vi "read_attributes.vi"(8 "error in (no error)":errorcluster, 11 "SVC in":refnum<class "SVC.lvclass">) -> (0 "error out":errorcluster, 2 "attributes":T1, 3 "SVC out":refnum<class "SVC.lvclass">)   [LabVIEW 2020, in "SVC.lvclass"]
uses:
  SVC.lvclass
  Controls/svc_attributes.ctl
  SVC.lvclass/SVC.ctl
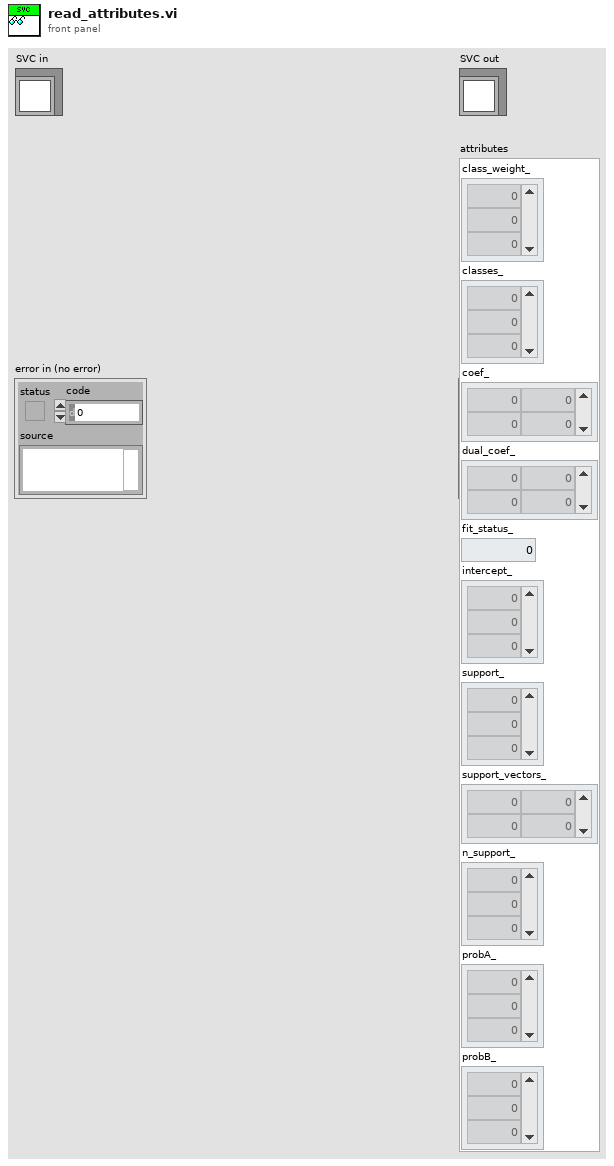
[diagram p1: front panel]
types:
  T1 = typedef "svc_attributes.ctl" = cluster{"class_weight_":dbl[], "classes_":dbl[], "coef_":dbl[][], "dual_coef_":dbl[][], "fit_status_":dbl, "intercept_":dbl[], "support_":dbl[], "support_vectors_":dbl[][], "n_support_":dbl[], "probA_":dbl[], "probB_":dbl[]}
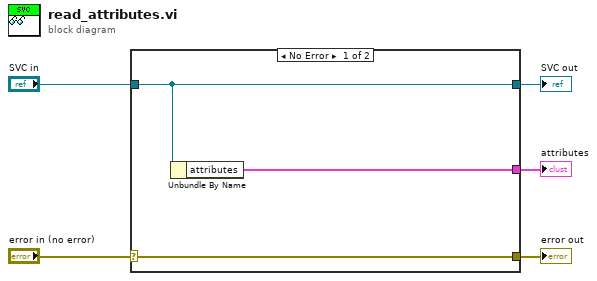
[diagram p0: block diagram]
diagram:
  n1 = case shown="No Error" "error in (no error)" {
    selector: "error in (no error)" -> [w8 w9]
    tunnel: [w8 w9] -> w4
    tunnel: [w7 w10] -> w2
    tunnel: "SVC in" -> [w7 w10]
    tunnel: [w6 _] -> w1
    frame No Error {
      n2 = Unbundle By Name(w7) -> ("attributes"=w6:T1)
    }
    frame Error {
    }
  }
  "error out" <- w4
  "SVC out" <- w2
  "attributes" <- w1
